vi "Pockels Cal-Generate cal conditions array.vi"() -> (3 "Pockels cal conditions array":string[][](array[string]))   [LabVIEW 2020]
uses:
  Globals/gl_Calibration globals.vi
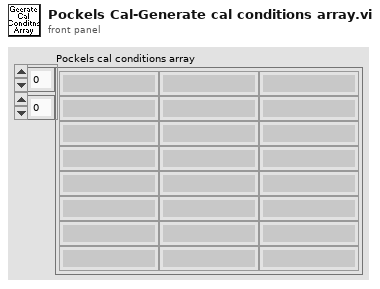
[diagram p1: front panel]
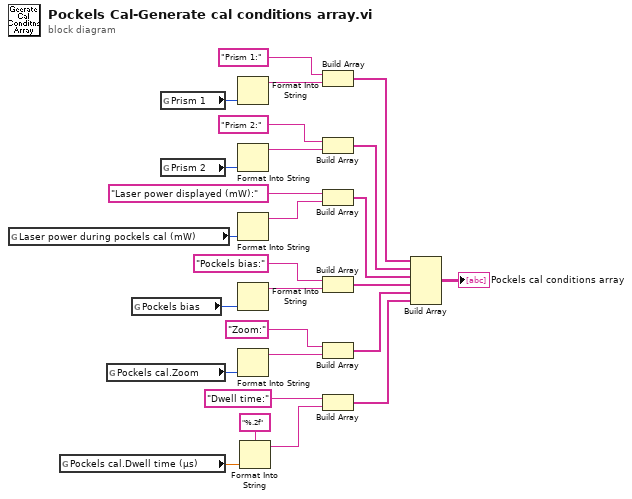
[diagram p0: block diagram]
diagram:
  n1 = global read "gl_Calibration globals.vi" "Laser power during pockels cal (mW)"() -> (w2:u16)
  n2 = global read "gl_Calibration globals.vi" "Pockels cal.Dwell time (µs)"() -> (w7:dbl)
  n3 = global read "gl_Calibration globals.vi" "Pockels cal.Zoom"() -> (w5:u8)
  n4 = global read "gl_Calibration globals.vi" "Pockels bias"() -> (w20:i16)
  n5 = global read "gl_Calibration globals.vi" "Prism 1"() -> (w14:u16)
  n6 = global read "gl_Calibration globals.vi" "Prism 2"() -> (w15:u16)
  n7 = Format Into String(w14) -> (resulting string=w12:string)  [unwired: 3 in, 1 out]
  n8 = Format Into String(w15) -> (resulting string=w17:string)  [unwired: 3 in, 1 out]
  n9 = Format Into String(w2) -> (resulting string=w4:string)  [unwired: 3 in, 1 out]
  n10 = Format Into String(w20) -> (resulting string=w18:string)  [unwired: 3 in, 1 out]
  n11 = Format Into String(w5) -> (resulting string=w11:string)  [unwired: 3 in, 1 out]
  n12 = Format Into String(format string="%.2f", w7) -> (resulting string=w8:string)  [unwired: 2 in, 1 out]
  n13 = Build Array("Prism 1:" ("format string"), w12) -> (w21:string[])
  n14 = Build Array("Prism 2:" ("format string"), w17) -> (w22:string[])
  n15 = Build Array("Laser power displayed (mW):" ("format string"), w4) -> (w1:string[])
  n16 = Build Array("Pockels bias:" ("format string"), w18) -> (w23:string[])
  n17 = Build Array("Zoom:" ("format string"), w11) -> (w24:string[])
  n18 = Build Array("Dwell time:" ("format string"), w8) -> (w25:string[])
  n19 = Build Array(w21, w22, w1, w23, w24, w25) -> (→"Pockels cal conditions array":string[][])
